vi "Launch.vi"() -> ()   [LabVIEW 2021, in "CIFCorePlugin.lvlib"]
uses:
  CIFCorePlugin.lvlib
  Class/CIFCorePlugin.lvclass
  Class/CIFCorePlugin.lvclass/CIFCorePlugin.ctl
  CIFUtilities/CIFLogs/CIFLogs.lvlib
panel:
  out "gRPC Server Port":i32
  in  "Plugin Name":string="Plugin Name Here"
  in  "host ip":string="localhost"
  in  "port":u16=1256
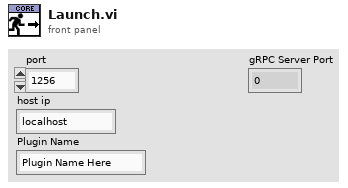
[diagram p1: front panel]
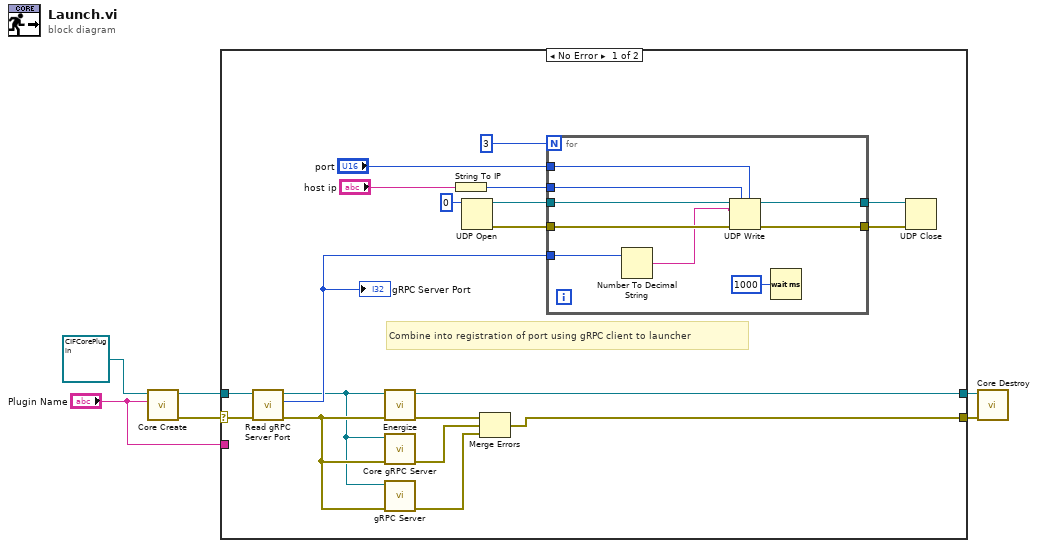
[diagram p0: block diagram]
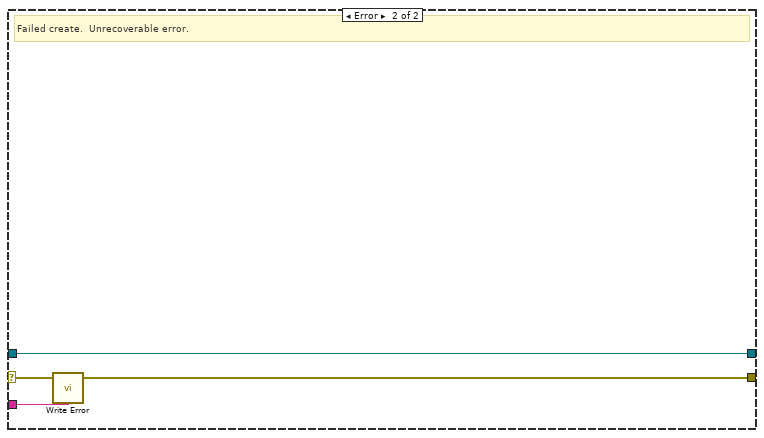
[diagram p2: hidden frame]
diagram:
  n1 = call "Core Create.vi"("Plugin Name"="Plugin Name", "CIFTemplateNode in"=refnum<class "CIFCorePlugin.lvclass"> refnum ("CIFCorePlugin.lvclass")) -> ("error out"=w3:errorcluster, "CIFTemplateNode out"=w5:refnum<class "CIFCorePlugin.lvclass">)  [unwired: 8 in]
  n2 = case shown="No Error" w3 {
    selector: w3 -> [w16 w38]
    tunnel: [w24 w35] -> w6
    tunnel: w5 -> [w22 w35]
    tunnel: [w18 w36] -> w4
    tunnel: "Plugin Name" -> [_ w37]
    frame No Error {
      # "Combine into registration of port using gRPC client to launcher"
      n3 = call "Read gRPC Server Port.vi"("error in (no error)"=w16, "CIFTemplateNode in"=w22) -> ("error out"=w23:errorcluster, "gRPC Server Port"=w25:i32, "CIFTemplateNode out"=w17:refnum<class "CIFCorePlugin.lvclass">)  [unwired: 7 in]
      "gRPC Server Port" <- w25
      n4 = call "Energize.vi"("error in (no error)"=w23, "CIFCorePlugin in"=w17) -> ("error out"=w21:errorcluster, "CIFCorePlugin out"=w24:refnum<class "CIFCorePlugin.lvclass">)  [unwired: 8 in]
      n5 = call "Core gRPC Server.vi"("error in (no error)"=w23, "CIFTemplateNode in"=w17) -> ("error out"=w20:errorcluster)  [unwired: 8 in, 1 out]
      n6 = call-dynamic "gRPC Server.vi"("error in (no error)"=w23, "CIFTemplateNode in"=w17) -> ("error out"=w19:errorcluster)  [unwired: 8 in, 1 out]
      n7 = String To IP(1:"host ip") -> (0:w12:u32)
      n8 = UDP Open(11:u16 0 ("port")) -> (port=w9:refnum<k16>, 0:w10:errorcluster)  [unwired: 4 in, 1 out]
      n9 = Merge Errors(w21, w20, w19) -> (w18:errorcluster)
      n10 = for {
        N: 3 -> [_]
        tunnel: w9 -> [w34]
        tunnel: w10 -> [w33]
        tunnel: "port" -> [w32]
        tunnel: w12 -> [w31]
        tunnel: [w28] -> w14
        tunnel: [w27] -> w15
        tunnel: w25 -> [w26]
        n11 = Number To Decimal String(number=w26) -> (decimal integer string=w29:string)  [unwired: 1 in]
        n12 = UDP Write(address=w31, port or service name=w32, connection ID=w34, data in=w29, 8:w33) -> (error out=w27:errorcluster, 3:w28:refnum<k16>)  [unwired: 1 in]
        n13 = Wait (ms)(milliseconds to wait=u32 1000) -> ()  [unwired: 1 out]
      }
      n14 = UDP Close(connection ID=w14, 8:w15) -> ()  [unwired: 2 out]
    }
    frame Error {
      # "Failed create.  Unrecoverable error."
      n15 = call "Write Error.vi"("error in (no error)"=w38, "Plugin Name"=w37) -> ("cleared error"=w36:errorcluster)  [unwired: 2 in]
    }
  }
  n16 = call "Core Destroy.vi"("error in (no error)"=w4, "CIFTemplateNode in"=w6) -> ()  [unwired: 8 in, 2 out]
